vi "_Subsystem_Name Controller Interactive Check.vi"(8 "Interactive Command in":T1, 9 "Default Command":T1, 11 "Buttons":cluster{"Execute Cmd":bool, "Abort Cmd":bool}) -> (1 "Interactive Command out":T1, 2 "Trace String":string, 3 "Schedule":bool)   [LabVIEW 2017]
doc: "Check the Execute and Abort buttons and choose the data and trace string."
uses:
  _Subsystem_Name Setpoints.ctl
  _Subsystem_Name Operations.ctl
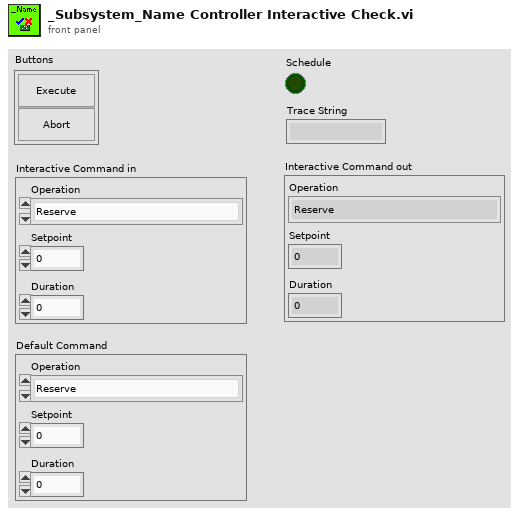
[diagram p1: front panel]
types:
  T1 = typedef "_Subsystem_Name Setpoints.ctl" = cluster{"Operation":T2, "Setpoint":dbl, "Duration":dbl}
  T2 = typedef "_Subsystem_Name Operations.ctl" = enum16{"Reserve", "Read Current", "Immediate"}
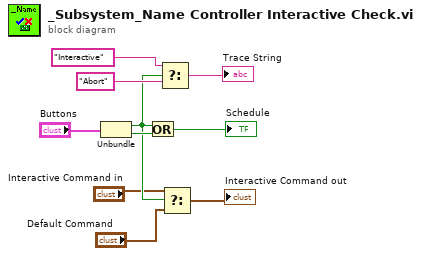
[diagram p0: block diagram]
diagram:
  n1 = Unbundle("Buttons") -> ("Execute Cmd"=w6:bool, "Abort Cmd"=w7:bool)
  n2 = Or(x=w6, y=w7) -> (x .or. y?=→"Schedule":bool)
  n3 = Select(t="Interactive", s=w6, f="Abort") -> (s? t:f=→"Trace String":string)
  n4 = Select(t="Interactive Command in", s=w6, f="Default Command") -> (s? t:f=→"Interactive Command out":T1)
